vi "raw checksum.vi"(11 "Array":u8[](array[numeric])=[139, 242, 0, 160, 247, 0] format="%.0x") -> (0 "Checksum Error":bool, 1 "Array Output":u8[](array[numeric])=[139, 242, 0, 160, 247, 0] format="%.0x", 2 "Calculated Checksum8":u8 format="%.0x", 3 "Input Checksum8":u8 format="%.0x", 4 "Calculated Checksum16 MSB":u8 format="%.0x", 5 "Input Checksum16 MSB":u8 format="%.0x", 6 "Calculated Checksum16 LSB":u8 format="%.0x", 7 "Input Checksum16 LSB":u8 format="%.0x")   [LabVIEW 2020]
panel:
  # "Checksum8"
  # "Checksum16 MSB"
  # "Checksum16 LSB"
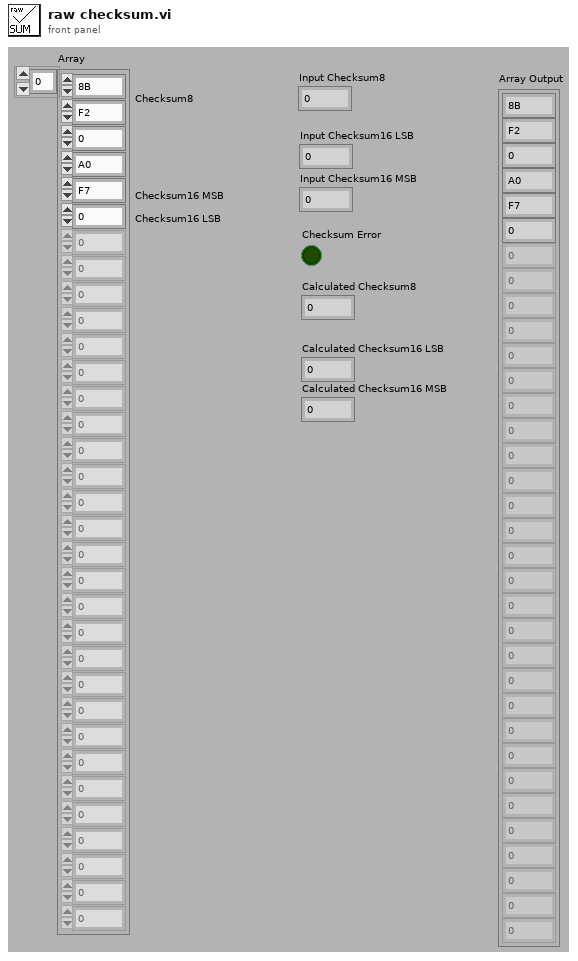
[diagram p1: front panel]
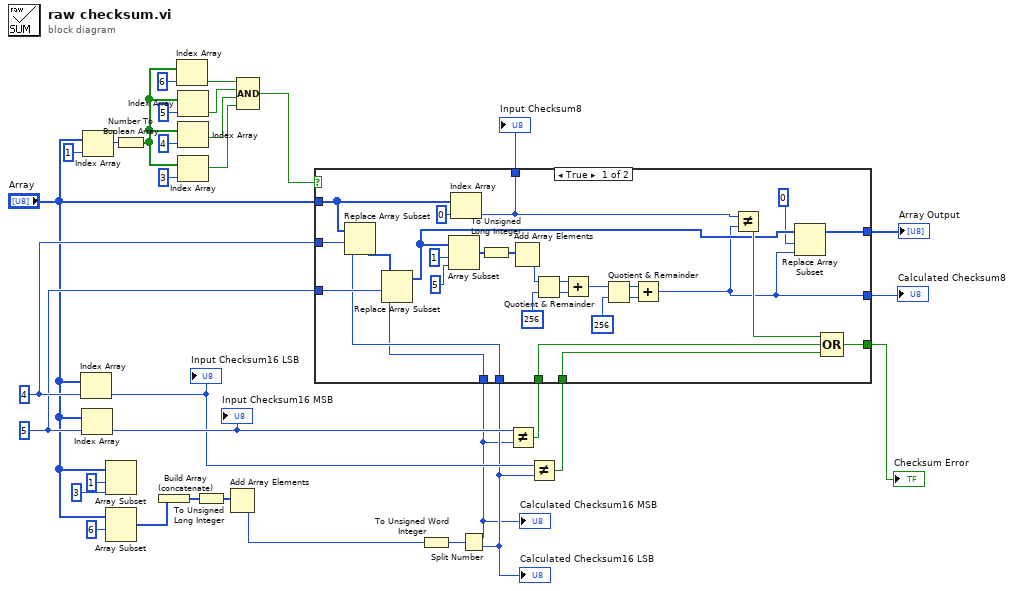
[diagram p0: block diagram]
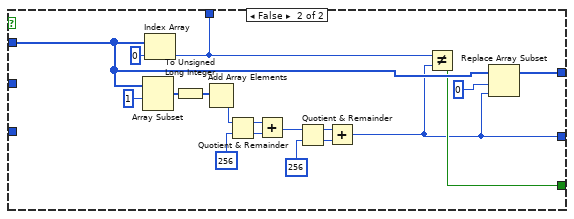
[diagram p2: hidden frame]
diagram:
  w21 = 5 ("Index")
  w22 = 4 ("Index")
  n1 = Index Array(array="Array", index=w22) -> (element=w26:u8)
  "Input Checksum16 LSB" <- w26
  n2 = Index Array(array="Array", index=w21) -> (element=w27:u8)
  "Input Checksum16 MSB" <- w27
  n3 = Index Array(array="Array", index=1 ("Index")) -> (element=w12:u8)
  n4 = Array Subset(array="Array", index=1 ("Array Index"), length=3 ("Array Length")) -> ()  [unwired: 1 out]
  n5 = Array Subset(array="Array", index=6 ("Array Index")) -> (w30:u8[])  [unwired: 1 in]
  n6 = Number To Boolean Array(number=w12) -> (Boolean array=w7:bool[])
  n7 = Build Array (concatenate)(w30) -> (w28:u8[])
  n8 = Index Array(array=w7, index=6 ("Index")) -> (element=w6:bool)
  n9 = Index Array(array=w7, index=5 ("Index")) -> (element=w5:bool)
  n10 = Index Array(array=w7, index=4 ("Index")) -> (element=w4:bool)
  n11 = Index Array(array=w7, index=3 ("Index")) -> (element=w3:bool)
  n12 = To Unsigned Long Integer(number=w28) -> (unsigned 32bit integer=w29:u32[])
  n13 = Add Array Elements(numeric array=w29) -> (sum=w1:u32)
  n14 = Compound Arithmetic op=AND(w6, w5, w4, w3) -> (w2:bool)
  n15 = To Unsigned Word Integer(number=w1) -> (unsigned 16bit integer=w15:u16)
  n16 = Split Number(x=w15) -> (hi(x)=w19:u8, lo(x)=w20:u8)
  "Calculated Checksum16 MSB" <- w19
  "Calculated Checksum16 LSB" <- w20
  n17 = Not Equal?(x=w27, y=w19) -> (x != y?=w25:bool)
  n18 = Not Equal?(x=w26, y=w20) -> (x != y?=w24:bool)
  n19 = case shown="True" w2 {
    tunnel: w25 -> [w53 _]
    tunnel: w24 -> [w52 _]
    tunnel: [w51 w68] -> w23
    tunnel: "Array" -> [w49 w69]
    tunnel: w22 -> [w48 _]
    tunnel: w21 -> [w47 _]
    tunnel: w20 -> [w46 _]
    tunnel: w19 -> [w45 _]
    tunnel: [w44 w71] -> w18
    tunnel: [w42 w70] -> w17
    tunnel: [w35 w63] -> w16
    frame True {
      n20 = Replace Array Subset(array=w49, new element=w46, index=w48) -> (w50:u8[])
      n21 = Replace Array Subset(array=w50, new element=w45, index=w47) -> (w41:u8[])
      n22 = Array Subset(array=w41, index=1 ("Array Index"), length=5 ("Array Length")) -> (w55:u8[])
      n23 = Index Array(array=w49, index=0 ("Index")) -> (element=w42:u8)
      n24 = To Unsigned Long Integer(number=w55) -> (unsigned 32bit integer=w54:u32[])
      n25 = Add Array Elements(numeric array=w54) -> (sum=w57:u32)
      n26 = Quotient & Remainder(x=w57, y=u16 256) -> (x-y*floor(x/y)=w60:u32, floor(x/y)=w59:u32)
      n27 = Add(x=w60, y=w59) -> (x+y=w36:u32)
      n28 = Quotient & Remainder(x=w36, y=u16 256) -> (x-y*floor(x/y)=w38:u32, floor(x/y)=w37:u32)
      n29 = Add(x=w38, y=w37) -> (x+y=w35:u32)
      n30 = Not Equal?(x=w42, y=w35) -> (x != y?=w43:bool)
      n31 = Replace Array Subset(array=w41, new element=w35, index=0 ("Index")) -> (w44:u8[])
      n32 = Compound Arithmetic op=OR(w43, w53, w52) -> (w51:bool)
    }
    frame False {
      n33 = Array Subset(array=w69, index=1 ("Array Index")) -> (w73:u8[])  [unwired: 1 in]
      n34 = Index Array(array=w69, index=0 ("Index")) -> (element=w70:u8)
      n35 = To Unsigned Long Integer(number=w73) -> (unsigned 32bit integer=w72:u32[])
      n36 = Add Array Elements(numeric array=w72) -> (sum=w75:u32)
      n37 = Quotient & Remainder(x=w75, y=u16 256) -> (x-y*floor(x/y)=w78:u32, floor(x/y)=w77:u32)
      n38 = Add(x=w78, y=w77) -> (x+y=w64:u32)
      n39 = Quotient & Remainder(x=w64, y=u16 256) -> (x-y*floor(x/y)=w66:u32, floor(x/y)=w65:u32)
      n40 = Add(x=w66, y=w65) -> (x+y=w63:u32)
      n41 = Not Equal?(x=w70, y=w63) -> (x != y?=w68:bool)
      n42 = Replace Array Subset(array=w69, new element=w63, index=0 ("Index")) -> (w71:u8[])
    }
  }
  "Calculated Checksum8" <- w16
  "Input Checksum8" <- w17
  "Checksum Error" <- w23
  "Array Output" <- w18
